vi "Rcalc.vi"(1 "roll":dbl=0.088, 2 "pitch":dbl=0.115) -> (0 "appended array":T1)   [LabVIEW 2019]
uses:
  <vilib>/Analysis/Matrix/Datatypes/RealMatrix.ctl
  <vilib>/Analysis/Matrix/NI_Matrix.lvlib
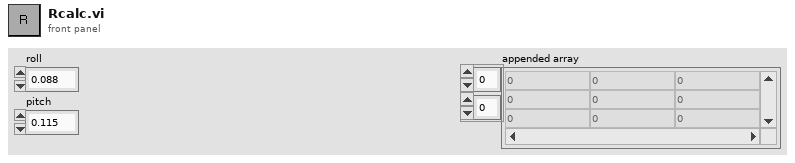
[diagram p1: front panel]
types:
  T1 = typedef "NI_Matrix.lvlib/RealMatrix.ctl" = dbl[][]
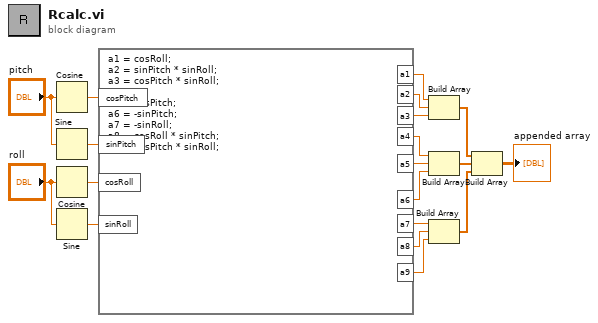
[diagram p0: block diagram]
diagram:
  n1 = Cosine(x="pitch") -> (cos(x)=w17:dbl)
  n2 = Sine(x="pitch") -> (sin(x)=w16:dbl)
  n3 = Cosine(x="roll") -> (cos(x)=w15:dbl)
  n4 = Sine(x="roll") -> (sin(x)=w14:dbl)
  n5 = formula code="a1 = cosRoll;\na2 = sinPitch * sinRoll;\na3 = cosPitch * sinRoll;\na4 = 0;\na5 = cosPitch;\na6 = -sinPitch;\na7 = -sinRoll;\na8 = cosRoll * sinPitch;\na9 = cosPitch * sinRoll;"("cosPitch"=w17, "sinPitch"=w16, "cosRoll"=w15, "sinRoll"=w14) -> ("a1"=w13:dbl, "a2"=w12:dbl, "a3"=w11:dbl, "a4"=w10:dbl, "a5"=w9:dbl, "a6"=w8:dbl, "a7"=w7:dbl, "a8"=w6:dbl, "a9"=w5:dbl)
  n6 = Build Array(w13, w12, w11) -> (w4:dbl[])
  n7 = Build Array(w10, w9, w8) -> (w3:dbl[])
  n8 = Build Array(w7, w6, w5) -> (w2:dbl[])
  n9 = Build Array(w4, w3, w2) -> (→"appended array":T1)
